vi "Get Installed SR Type.vi"(8 "error in (no error)":errorcluster, 11 "VISA Refnum in":refnum<visa-resource-name>="COM1") -> (0 "error out":errorcluster, 2 "SR":string, 3 "VISA Refnum out":refnum<visa-resource-name>)   [LabVIEW 2019, in "KH7008.lvlib"]
uses:
  KH7008.lvlib
  typedefs/shunt--enum.ctl
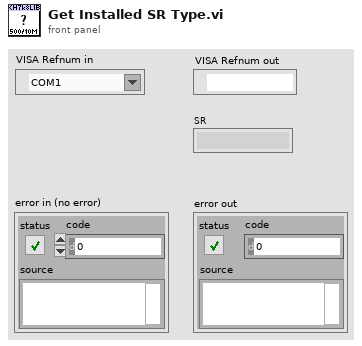
[diagram p1: front panel]
types:
  T1 = typedef "KH7008.lvlib/shunt--enum.ctl" = enum16{"Open", "50", "500", "5k", "50k", "10M"}
  T2 = typedef "KH7008.lvlib/allChannelProperties--Array.ctl" = T3[]
  T3 = typedef "KH7008.lvlib/channelProperties--Cluster.ctl" = cluster{"channel":T4, "gain":T5, "input":T6, "shunt":T1, "couple":T7, "filter":T8}
  T4 = typedef "KH7008.lvlib/channel--numeric.ctl" = u16
  T5 = typedef "KH7008.lvlib/gain--enum.ctl" = enum16{"1", "10", "100", "1000"}
  T6 = typedef "KH7008.lvlib/input--enum.ctl" = enum16{"OFF", "SE+", "SE-", "DIFF"}
  T7 = typedef "KH7008.lvlib/couple--enum.ctl" = enum16{"AC", "DC"}
  T8 = typedef "KH7008.lvlib/filter--enum.ctl" = enum16{"OFF", "ON"}
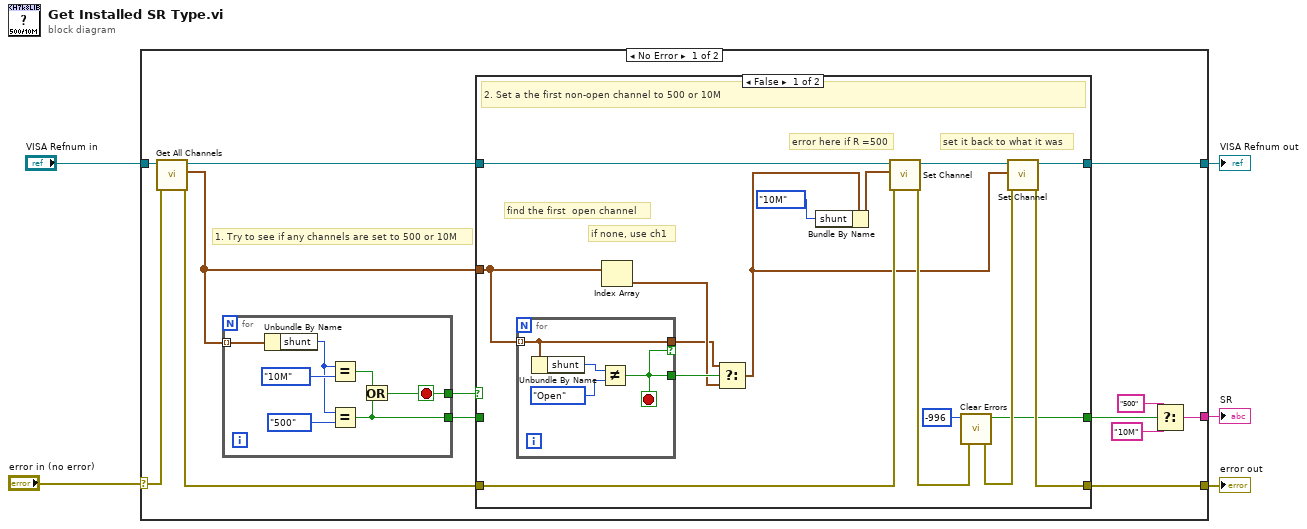
[diagram p0: block diagram]
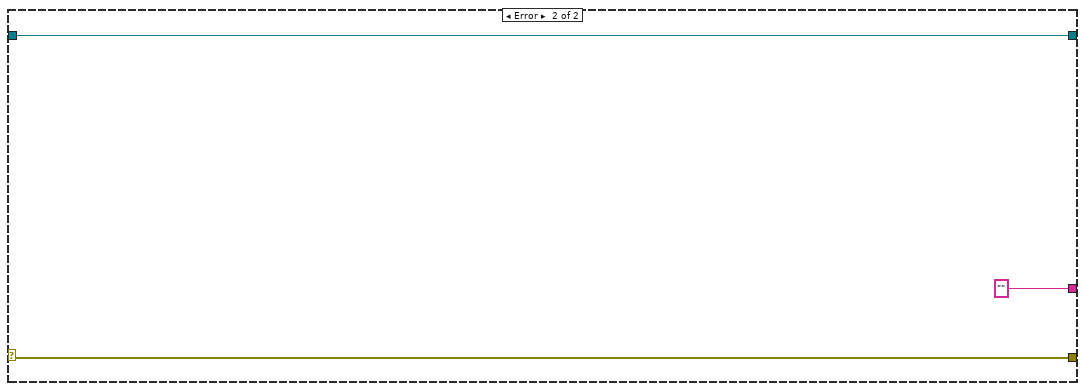
[diagram p3: hidden frame]
diagram:
  n1 = case shown="No Error" "error in (no error)" {
    selector: "error in (no error)" -> [w17 w49]
    tunnel: "VISA Refnum in" -> [w18 w51]
    tunnel: [w10 w51] -> w3
    tunnel: [w9 ""] -> w2
    tunnel: [w8 w49] -> w1
    frame No Error {
      # "1. Try to see if any channels are set to 500 or 10M"
      n2 = call "Get All Channels.vi"("error in (no error)"=w17, "VISA Refnum in"=w18) -> ("error out"=w16:errorcluster, "allChannelProperties"=w13:T2, "VISA Refnum out"=w14:refnum<visa-resource-name>)  [unwired: 7 in]
      n3 = for {
        tunnel: w13 -> [w25] mode=indexing
        tunnel: [w20] -> w15
        tunnel: [w19] -> w12
        stop <- w20 stop-if-true
        n4 = Unbundle By Name(w25) -> ("shunt"=w22:T1)
        n5 = Equal?(x=w22, y=shunt--enum."10M" ("shunt")) -> (x = y?=w21:bool)
        n6 = Equal?(x=w22, y=shunt--enum."500" ("shunt")) -> (x = y?=w19:bool)
        n7 = Or(x=w21, y=w19) -> (x .or. y?=w20:bool)
      }
      n8 = case shown="False" w15 {
        tunnel: w16 -> [w39 w46]
        tunnel: w14 -> [w41 w47]
        tunnel: w13 -> [w30 _]
        tunnel: w12 -> [_ w48]
        tunnel: [w32 w48] -> w11
        tunnel: [w34 w47] -> w10
        tunnel: [w33 w46] -> w8
        frame False {
          # "if none, use ch1"
          # "find the first  open channel"
          # "set it back to what it was"
          # "error here if R =500"
          # "2. Set a the first non-open channel to 500 or 10M"
          n9 = for {
            tunnel: w30 -> [w43] mode=indexing
            tunnel: [w43] -> w26 if=w42
            tunnel: [w42] -> w29
            stop <- w42 stop-if-true
            n10 = Unbundle By Name(w43) -> ("shunt"=w45:T1)
            n11 = Not Equal?(x=w45, y=shunt--enum."Open" ("shunt")) -> (x != y?=w42:bool)
          }
          n12 = Index Array(array=w30) -> (element=w28:T3)  [unwired: 1 in]
          n13 = Select(t=w26, s=w29, f=w28) -> (s? t:f=w27:T3)
          n14 = Bundle By Name(cluster=w27, "shunt"=shunt--enum."10M") -> (w40:T3)
          n15 = call "Set Channel.vi"("error in (no error)"=w39, "channelParameter"=w40, "VISA Refnum in"=w41) -> ("error out"=w36:errorcluster, "VISA Refnum out"=w37:refnum<visa-resource-name>)  [unwired: 7 in]
          n16 = call <vilib>:"Clear Errors.vi"("error in (no error)"=w36, "specific error code to clear (0: all)"=-996) -> ("error out"=w35:errorcluster, "specific error cleared?"=w32:bool)  [unwired: 4 in]
          n17 = call "Set Channel.vi"("error in (no error)"=w35, "channelParameter"=w27, "VISA Refnum in"=w37) -> ("error out"=w33:errorcluster, "VISA Refnum out"=w34:refnum<visa-resource-name>)  [unwired: 7 in]
        }
        frame True {
          # "1.One of the channels was 500 or 10M"
        }
      }
      n18 = Select(t="500", s=w11, f="10M") -> (s? t:f=w9:string)
    }
    frame Error {
    }
  }
  "VISA Refnum out" <- w3
  "error out" <- w1
  "SR" <- w2
